vi "列表框取列数组.vi"(9 "列":i32, 11 "引用":refnum<vi>) -> (3 "列数组":string[](array[string]))   [LabVIEW 2016]
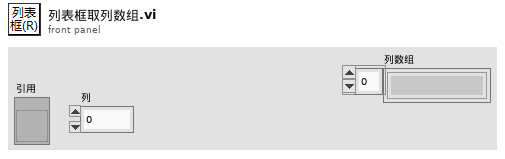
[diagram p1: front panel]
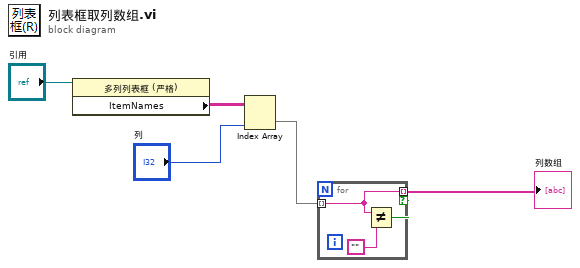
[diagram p0: block diagram]
diagram:
  n1 = property class="多列列表框 (严格)"(reference="引用") -> ("ItemNames"=w4:string[][])  [unwired: 1 in, 2 out]
  n2 = Index Array(array=w4, index (col)="列") -> (element=w2:string[])  [unwired: 1 in]
  n3 = for {
    tunnel: w2 -> [w7] mode=indexing
    tunnel: [w7] -> w1 mode=indexing if=w6
    n4 = Not Equal?(x=w7, y="") -> (x != y?=w6:bool)
  }
  "列数组" <- w1
